vi "Property Terminal_Unwired.vi"(8 "error in":errorcluster, 10 "Term Refnum":refnum<vi>, 11 "PropertyItem in":refnum<vi>) -> (0 "error out":errorcluster, 2 "Is Write":bool, 3 "Unwired":bool)   [LabVIEW 2023]
doc: "Returns true of a property terminal is unwired or the wire is broken.\n\nCan take a terminal reference or a property item reference."
panel:
  # "OR"
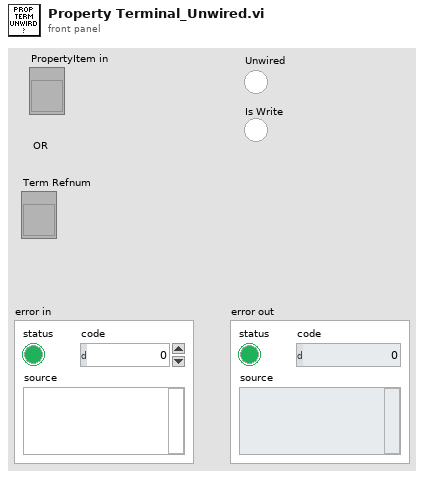
[diagram p1: front panel]
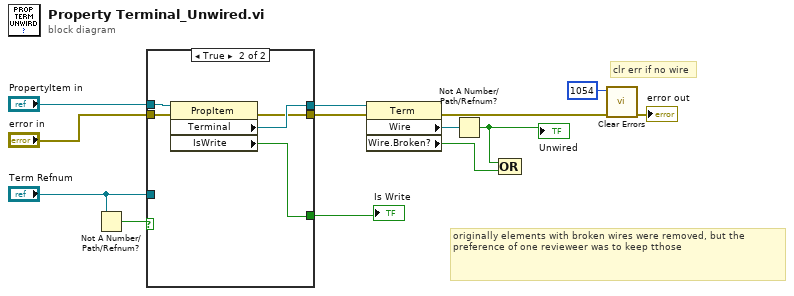
[diagram p0: block diagram]
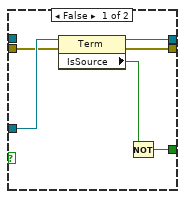
[diagram p2: hidden frame]
diagram:
  # "originally elements with broken wires were removed, but the preference of one revieweer was to keep tthose"
  # "clr err if no wire"
  n1 = Not A Number/Path/Refnum?(number/path/refnum="Term Refnum") -> (NaN/Path/Refnum?=w9:bool)
  n2 = case shown="True" w9 {
    tunnel: [w18 w24] -> w11
    tunnel: "PropertyItem in" -> [_ w23]
    tunnel: "Term Refnum" -> [w19 _]
    tunnel: [w16 w22] -> w4
    tunnel: "error in" -> [w15 w21]
    tunnel: [w14 w20] -> w2
    frame False {
      n3 = property class="Term"(reference=w19, error in=w15) -> (reference out=w18:refnum<vi>, error out=w14:errorcluster, "IsSource"=w17:bool)
      n4 = Not(x=w17) -> (.not. x?=w16:bool)
    }
    frame True {
      n5 = property class="PropItem"(reference=w23, error in=w21) -> (error out=w20:errorcluster, "Terminal"=w24:refnum<vi>, "IsWrite"=w22:bool)  [unwired: 1 out]
    }
  }
  "Is Write" <- w4
  n6 = property class="Term"(reference=w11, error in=w2) -> (error out=w7:errorcluster, "Wire"=w12:refnum<vi>, "Wire.Broken?"=w13:bool)  [unwired: 1 out]
  n7 = Not A Number/Path/Refnum?(number/path/refnum=w12) -> (NaN/Path/Refnum?=w1:bool)
  "Unwired" <- w1
  n8 = Compound Arithmetic op=OR(w1, w13) -> ()  [unwired: 1 out]
  n9 = call <vilib>:"Clear Errors.vi"("error in (no error)"=w7, "specific error code to clear (0: all)"=1054) -> ("error out"=→"error out":errorcluster)  [unwired: 4 in, 1 out]
